vi "TTL_single.vi"() -> ()   [LabVIEW 2020]
uses:
  istr.lib/Agilent 33XXX Series/Agilent 33XXX Series.lvlib
panel:
  in  "stop":bool
  in  "Wait at high (ms)":u32=1
  out "error out":errorcluster
  out "Status":bool
  in  "Pulse height (V)":dbl=1.0
  in  "VISA resource name":refnum<visa-resource-name>
  in  "Pulse":bool
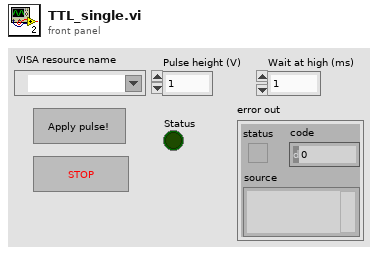
[diagram p1: front panel]
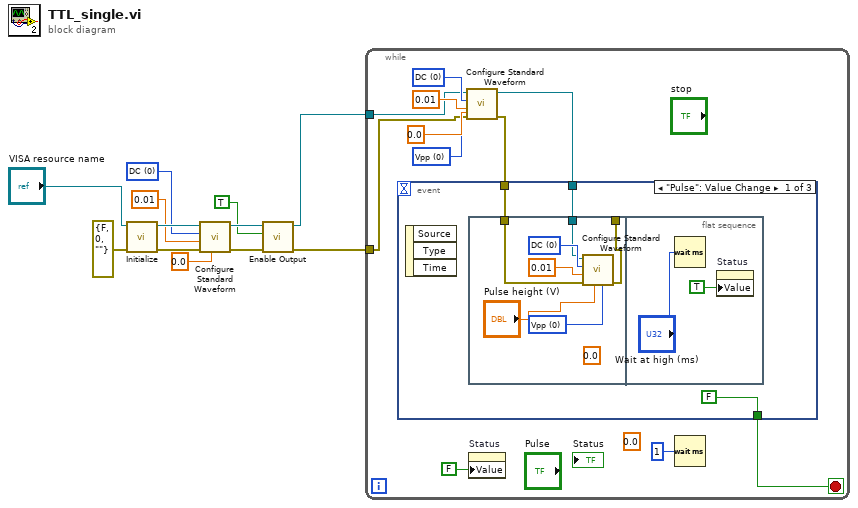
[diagram p0: block diagram]
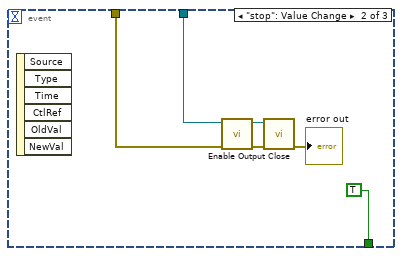
[diagram p2: hidden frame]
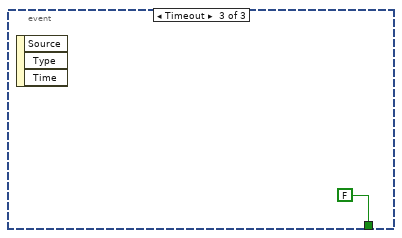
[diagram p3: hidden frame]
diagram:
  w8 = u16 0 items=["DC", "Sine", "Square", "Triangle", "Ramp", "Pulse", "Noise", "Sinc", "Negative Ramp", "Exponential Rise", "Exponential Fall", "Cardiac"] ("Waveform Function (1: Sine)")
  n1 = call "Initialize.vi"("error in (no error)"=errorcluster {"status"=FALSE, "code"=0, "source"=""}, "VISA resource name"="VISA resource name") -> ("error out"=w10:errorcluster, "VISA resource name out"=w11:refnum<visa-resource-name>)  [unwired: 8 in]
  n2 = call "Configure Standard Waveform.vi"("DC Offset (0.00 V)"=0.0, "error in (no error)"=w10, "Amplitude (1)"=0.01, "Waveform Function (1: Sine)"=w8, "VISA resource name"=w11) -> ("error out"=w4:errorcluster, "VISA resource name out"=w5:refnum<visa-resource-name>)  [unwired: 5 in]
  n3 = call "Enable Output.vi"("error in (no error)"=w4, "Enable Output  (T: Enable)"=TRUE, "VISA resource name"=w5) -> ("error out"=w1:errorcluster, "VISA resource name out"=w2:refnum<visa-resource-name>)  [unwired: 7 in]
  n4 = while {
    tunnel: w2 -> [w17]
    tunnel: w1 -> [w16]
    stop <- w13 stop-if-true
    (unwired) 0.0 ("DC Offset (0.00 V)")
    w19 = u16 0 items=["Vpp", "Vrms", "dB"] ("Unit (0: Vpp)")
    w21 = u16 0 items=["DC", "Sine", "Square", "Triangle", "Ramp", "Pulse", "Noise", "Sinc", "Negative Ramp", "Exponential Rise", "Exponential Fall", "Cardiac"] ("Waveform Function (1: Sine)")
    n5 = call "Configure Standard Waveform.vi"("Unit (0: Vpp)"=w19, "DC Offset (0.00 V)"=0.0, "error in (no error)"=w16, "Amplitude (1)"=0.01, "Waveform Function (1: Sine)"=w21, "VISA resource name"=w17) -> ("error out"=w15:errorcluster, "VISA resource name out"=w14:refnum<visa-resource-name>)  [unwired: 4 in]
    n6 = event shown="[0] \"Pulse\": Value Change" {
      selector: _ -> [_ _ _]
      dyn-events: _ -> [_ _ _]
      timeout: _ -> [_ _ _]
      tunnel: w15 -> [w26 w38 _]
      tunnel: w14 -> [w25 w37 _]
      tunnel: [FALSE TRUE FALSE] -> w13
      event "Pulse": Value Change {
        n7 = event-data() -> ()  [unwired: 1 in, 3 out]
        n8 = flat-sequence {
          tunnel: w26 -> [w30]
          tunnel: w25 -> [w29]
          tunnel: [w28] -> _
          frame #0 {
            (unwired) 0.0 ("DC Offset (0.00 V)")
            w33 = u16 0 items=["Vpp", "Vrms", "dB"] ("Unit (0: Vpp)")
            w32 = u16 0 items=["DC", "Sine", "Square", "Triangle", "Ramp", "Pulse", "Noise", "Sinc", "Negative Ramp", "Exponential Rise", "Exponential Fall", "Cardiac"] ("Waveform Function (1: Sine)")
            n9 = call "Configure Standard Waveform.vi"("Unit (0: Vpp)"=w33, "DC Offset (0.00 V)"="Pulse height (V)", "error in (no error)"=w30, "Amplitude (1)"=0.01, "Waveform Function (1: Sine)"=w32, "VISA resource name"=w29) -> ("error out"=w28:errorcluster)  [unwired: 4 in, 1 out]
          }
          frame #1 {
            n10 = Wait (ms)(milliseconds to wait="Wait at high (ms)") -> ()  [unwired: 1 out]
            n11 = property on="Status" class="Bool (strict)"("Value"=TRUE ("Enable Output  (T: Enable)")) -> ()  [unwired: 2 in, 2 out]
          }
        }
      }
      event "stop": Value Change {
        n12 = event-data() -> ()  [unwired: 1 in, 6 out]
        n13 = call "Enable Output.vi"("error in (no error)"=w38, "VISA resource name"=w37) -> ("error out"=w41:errorcluster, "VISA resource name out"=w40:refnum<visa-resource-name>)  [unwired: 8 in]
        n14 = call "Close.vi"("error in (no error)"=w41, "VISA resource name"=w40) -> ("error out"=→"error out":errorcluster)  [unwired: 9 in]
      }
      event Timeout {
        n15 = event-data() -> ()  [unwired: 1 in, 3 out]
      }
    }
    n16 = property on="Status" class="Bool (strict)"("Value"=FALSE ("Enable Output  (T: Enable)")) -> ()  [unwired: 2 in, 2 out]
    n17 = Wait (ms)(milliseconds to wait=u32 1) -> ()  [unwired: 1 out]
  }
